vi "Touch_Board.vi"() -> ()   [LabVIEW 2013]
uses:
  <resource>/objmgr/IMAQImage.rc
  <vilib>/vision/NI_Vision_Development_Module.lvlib
  User32.dll
  <vilib>/userdefined/High Color/IMAQdx.ctl
panel:
  in  "NEXT":bool
  in  "Boolean 2":bool
  out "x-y":sgl
  in  "Boolean":bool
  out "Increment":dbl
  in  "reset":i32(listbox)
  in  "Screen Resolution":cluster{"x":i32, "y":i32}={"x"=1366, "y"=768}
  out "Image Size":cluster{"x":i32, "y":i32}
  in  "stop":bool
  in  "Main Tab":enum32{"Page 1", "Page 2"}(tab)
  out "Image":T1(plugin-control)
  in  "Control Panel Tab":enum32{"Page 1", "Page 2", "Page 3"}(tab)
  out "Processed FPS":dbl(knob) scale=0.0..100.0
  out "Acquired FPS":dbl(knob) scale=0.0..100.0 scale format="%.1f"
  in  "Camera Name":T2="cam8"
  out "Buffer No.":u32=4294967295
  in  "Pulse":bool=TRUE
  in  "roi":bool
  in  "mask":bool
  in  "creat calib":bool
  in  "IR":bool
  in  "detect":bool
  in  "touch points":bool
  in  "open calib":bool
  in  "calc":bool=TRUE
  in  "cursor":bool=TRUE
  in  "Click":bool
  in  "Start":bool
  in  "Step":i32
  in  "Settings Tab":T3(tab)=enum."auto calib"
  in  "Prompt":string="Select The Rectangle - Screen Rregion"
  in  "Rectangle":T4 {"Rotation" format="%.2f"; "Left" scale=0.0..1024.0; "Right" scale=0.0..1024.0}
  in  "Color Palette":u32(colorbox)
  in  "ROI Descriptor":T5={"Global Rectangle"=[161, 85, 600, 422], "Contours"=[{"ID"=enum."External", "Type"=3, "Coordinates"=[161, 85, 600, 422]}]} {"Contours"."Type" items=["No Selection", "Point", "Line", "Rectangle", "Oval", "Polygon", "Free", "Annulus", "Unused2", "Unused3", "Broken Line", "Free Hand Line", "Rotated Rectangle"]}
  in  "Out / In":bool
  in  "Shrink":bool=TRUE
  out "Rect Array":i32[](array[numeric])
  in  "Camera Position":u16(ring)
  out "Q":dbl
  in  "Path":path=path "I:/Works/NI/Gesture/Touch Board/TB/cam.png"
  in  "Reference Points":T6 {"Unit" items=["Undefined", "Angstrom", "micrometer", "millimeter", "centimeter", "meter", "kilometer", "microinch", "inch", "feet", "nautic miles", "standard miles", "steps"]; "Real World Coordinates"."Y" format="%.2f"; "Real World Coordinates"."X" format="%.2f"; "Pixel Coordinates"."Y" format="%.2f"; "Pixel Coordinates"."X" format="%.2f"}
  in  "Calibration Axis Info":T7={"Origin Pixel"={"X"=0.0, "Y"=0.0}, "Angle Relative to Horizontal (deg)"=0.0, "Axis Reference"=1} {"Axis Reference" items=["Direct", "Indirect"]; "Angle Relative to Horizontal (deg)" format="%.2f"; "Origin Pixel"."Y" format="%.2f"; "Origin Pixel"."X" format="%.2f"}
  in  "Calibration Learn Setup":T8 {"Corrected Image Learn ROI" items=["Full Image ", "Calibration ROI", "ROI", "Calibration AND ROI", "Calibration OR ROI"]; "Corrected Image Scaling" items=["Scale to Preserve Area", "Scale to Fit"]; "Distortion" items=["Perspective", "Nonlinear"]}
  in  "Point":dbl
  out "Screen Points":T9={"R1"={"x"=0, "y"=0}, "R2"={"x"=1365, "y"=0}, "R3"={"x"=1365, "y"=767}, "R4"={"x"=0, "y"=767}}
  in  "R4":cluster{"x":i32, "y":i32}={"x"=0, "y"=767}
  in  "R3":cluster{"x":i32, "y":i32}={"x"=1365, "y"=767}
  in  "R2":cluster{"x":i32, "y":i32}={"x"=1365, "y"=0}
  in  "R1":cluster{"x":i32, "y":i32}
  in  "Path 2":path=path "I:/Works/NI/Gesture/Touch Board/TB/cam.png"
  in  "Interpolation Type":u32(ring)=1 items=["Zero Order", "Bi-Linear", "Quadratic", "Cubic Spline"]
  in  "Color Plane":i32(ring) items=["Red", "Green", "Blue", "Hue", "Saturation", "Luminance", "Value", "Intensity"]
  in  "Low Pass/High Pass (Low)":bool
  in  "Square/Hexa (Square)":bool
  in  "Connectivity 4/8 (8)":bool=TRUE
  in  "Number of Erosion":i32=1
  in  "Range":cluster{"Lower value":sgl, "Upper value":sgl}={"Lower value"=80.78014, "Upper value"=255.0} {"Lower value" scale=0.0..255.0; "Upper value" scale=0.0..255.0}
  in  "Connectivity 4/8 (8) 2":bool=TRUE
  out "Detect?":bool
  in  "ROI Side":T10={"Global Rectangle"=[0], "Contours"=[{"ID"=enum."External", "Type"=3, "Coordinates"=[]}]} {"Contours"."Type" items=["No Selection", "Point", "Line", "Rectangle", "Oval", "Polygon", "Freehand Region", "Annulus", "Unused2", "Unused3", "Broken Line", "Freehand Line", "Rotated Rectangle"]}
  in  "Settings S":T11={"Contrast"=1, "Filter width"=4, "Steepness"=2, "Subsampling Ratio"=5, "Show Search Area"=TRUE, "Show Search Lines"=TRUE, "Show Edges Found"=TRUE, "Show Result"=TRUE}
  in  "Settings T":T11={"Contrast"=1, "Filter width"=4, "Steepness"=2, "Subsampling Ratio"=5, "Show Search Area"=TRUE, "Show Search Lines"=TRUE, "Show Edges Found"=TRUE, "Show Result"=TRUE}
  out "Distance T":sgl format="%.2f"
  out "Distance S":sgl format="%.2f"
  in  "ROI Top":T10={"Global Rectangle"=[], "Contours"=[{"ID"=enum."External", "Type"=3, "Coordinates"=[]}]} {"Contours"."Type" items=["No Selection", "Point", "Line", "Rectangle", "Oval", "Polygon", "Freehand Region", "Annulus", "Unused2", "Unused3", "Broken Line", "Freehand Line", "Rotated Rectangle"]}
  out "Points of Contact T":cluster{"X":sgl, "Y":sgl}[](array[cluster]) {"Y" format="%.2f"; "X" format="%.2f"}
  out "Points of Contact S":cluster{"X":sgl, "Y":sgl}[](array[cluster]) {"Y" format="%.2f"; "X" format="%.2f"}
  in  "Scanning axis S":u32(ring) items=["Horizontal", "Vertical"]
  in  "Scanning axis T":u32(ring)=1 items=["Horizontal", "Vertical"]
  out "Centre":cluster{"X":sgl, "Y":sgl}
  out "Object Origin":cluster{"X":sgl, "Y":sgl}
  in  "Kx":dbl
  in  "Ky":dbl
  in  "C4":cluster{"x":i16, "y":i16}
  in  "C3":cluster{"x":i16, "y":i16}
  in  "C2":cluster{"x":i16, "y":i16}
  in  "C1":cluster{"x":i16, "y":i16}
  in  "Shift Origin":dbl
  out "Original":bool
  in  "Pulse Width":u32=50
  out "Delay":bool
  out "Stop Pulse":bool
  out "Start Pulse":bool
  in  "Screen Origin":cluster{"x":i16, "y":i16}
  out "M X":dbl
  out "M Y":dbl
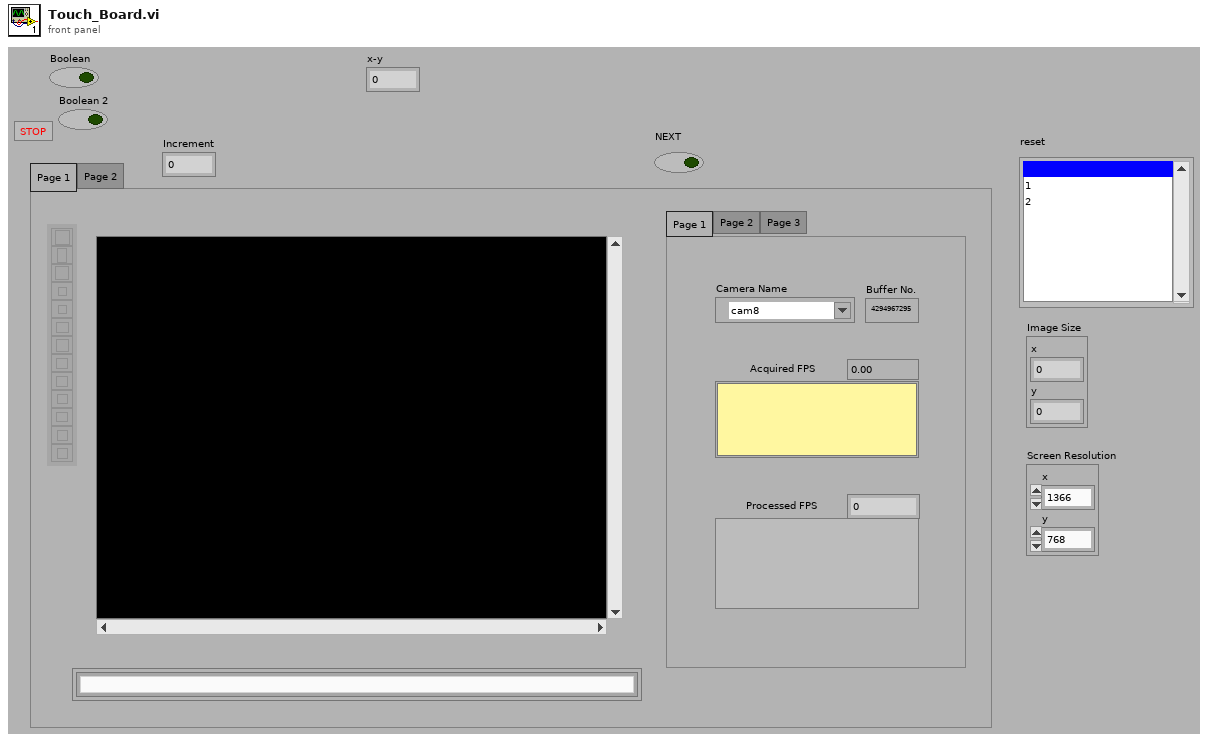
[diagram p1: front panel]
types:
  T1 = typedef "IMAQ Image.ctl" = refnum<image>
  T2 = typedef "IMAQdx.ctl" = refnum<k21>
  T3 = enum32{"rect", "mask", "creat calib", "open calib", "image process", "detect", "calc", "pulse", "Cursor", "auto calib"}
  T4 = typedef "IMAQ Rectangle" = cluster{"Left":i32, "Top":i32, "Right":i32, "Bottom":i32, "Rotation":dbl}
  T5 = cluster{"Global Rectangle":i32[], "Contours":cluster{"ID":enum32{"External", "Internal"}, "Type":u32, "Coordinates":i32[]}[]}
  T6 = cluster{"Pixel Coordinates":cluster{"X":sgl, "Y":sgl}[], "Real World Coordinates":cluster{"X":sgl, "Y":sgl}[], "Unit":u32}
  T7 = cluster{"Origin Pixel":cluster{"X":sgl, "Y":sgl}, "Angle Relative to Horizontal (deg)":sgl, "Axis Reference":u32}
  T8 = cluster{"Distortion":sgl, "Corrected Image Scaling":sgl, "Corrected Image Learn ROI":sgl, "Learn Error Map?":bool, "Learn Correction Table?":bool}
  T9 = cluster{"R1":cluster{"x":i16, "y":i16}, "R2":cluster{"x":i16, "y":i16}, "R3":cluster{"x":i16, "y":i16}, "R4":cluster{"x":i16, "y":i16}}
  T10 = typedef "ROI Descriptor" = cluster{"Global Rectangle":i32[], "Contours":cluster{"ID":enum32{"External", "Internal"}, "Type":u32, "Coordinates":i32[]}[]}
  T11 = cluster{"Contrast":i32, "Filter width":i32, "Steepness":i32, "Subsampling Ratio":u32, "Show Search Area":bool, "Show Search Lines":bool, "Show Edges Found":bool, "Show Result":bool}
  T12 = cluster{"Left":i32, "Top":i32, "Right":i32, "Bottom":i32}
  T13 = cluster{"Height":i32, "Height":i32, "x":i32, "y":i32}
  T14 = cluster{"R1":cluster{"x":i32, "y":i32}, "R2":cluster{"x":i32, "y":i32}, "R3":cluster{"x":i32, "y":i32}, "R4":cluster{"x":i32, "y":i32}}
  T15 = cluster{"Value":cluster{"x":i32, "y":i32}, cluster{"x":i32, "y":i32}, "Value":cluster{"x":i32, "y":i32}, "Value":cluster{"x":i32, "y":i32}}
  T16 = cluster{"Angles (deg)[0]":sgl, "Angles (deg)[1]":sgl, "Angles (deg)[2]":sgl, "Angles (deg)[3]":sgl, "Angles (deg)[4]":sgl, "Angles (deg)[5]":sgl, "Angles (deg)[6]":sgl, "Angles (deg)[7]":sgl, "Angles (deg)[8]":sgl}
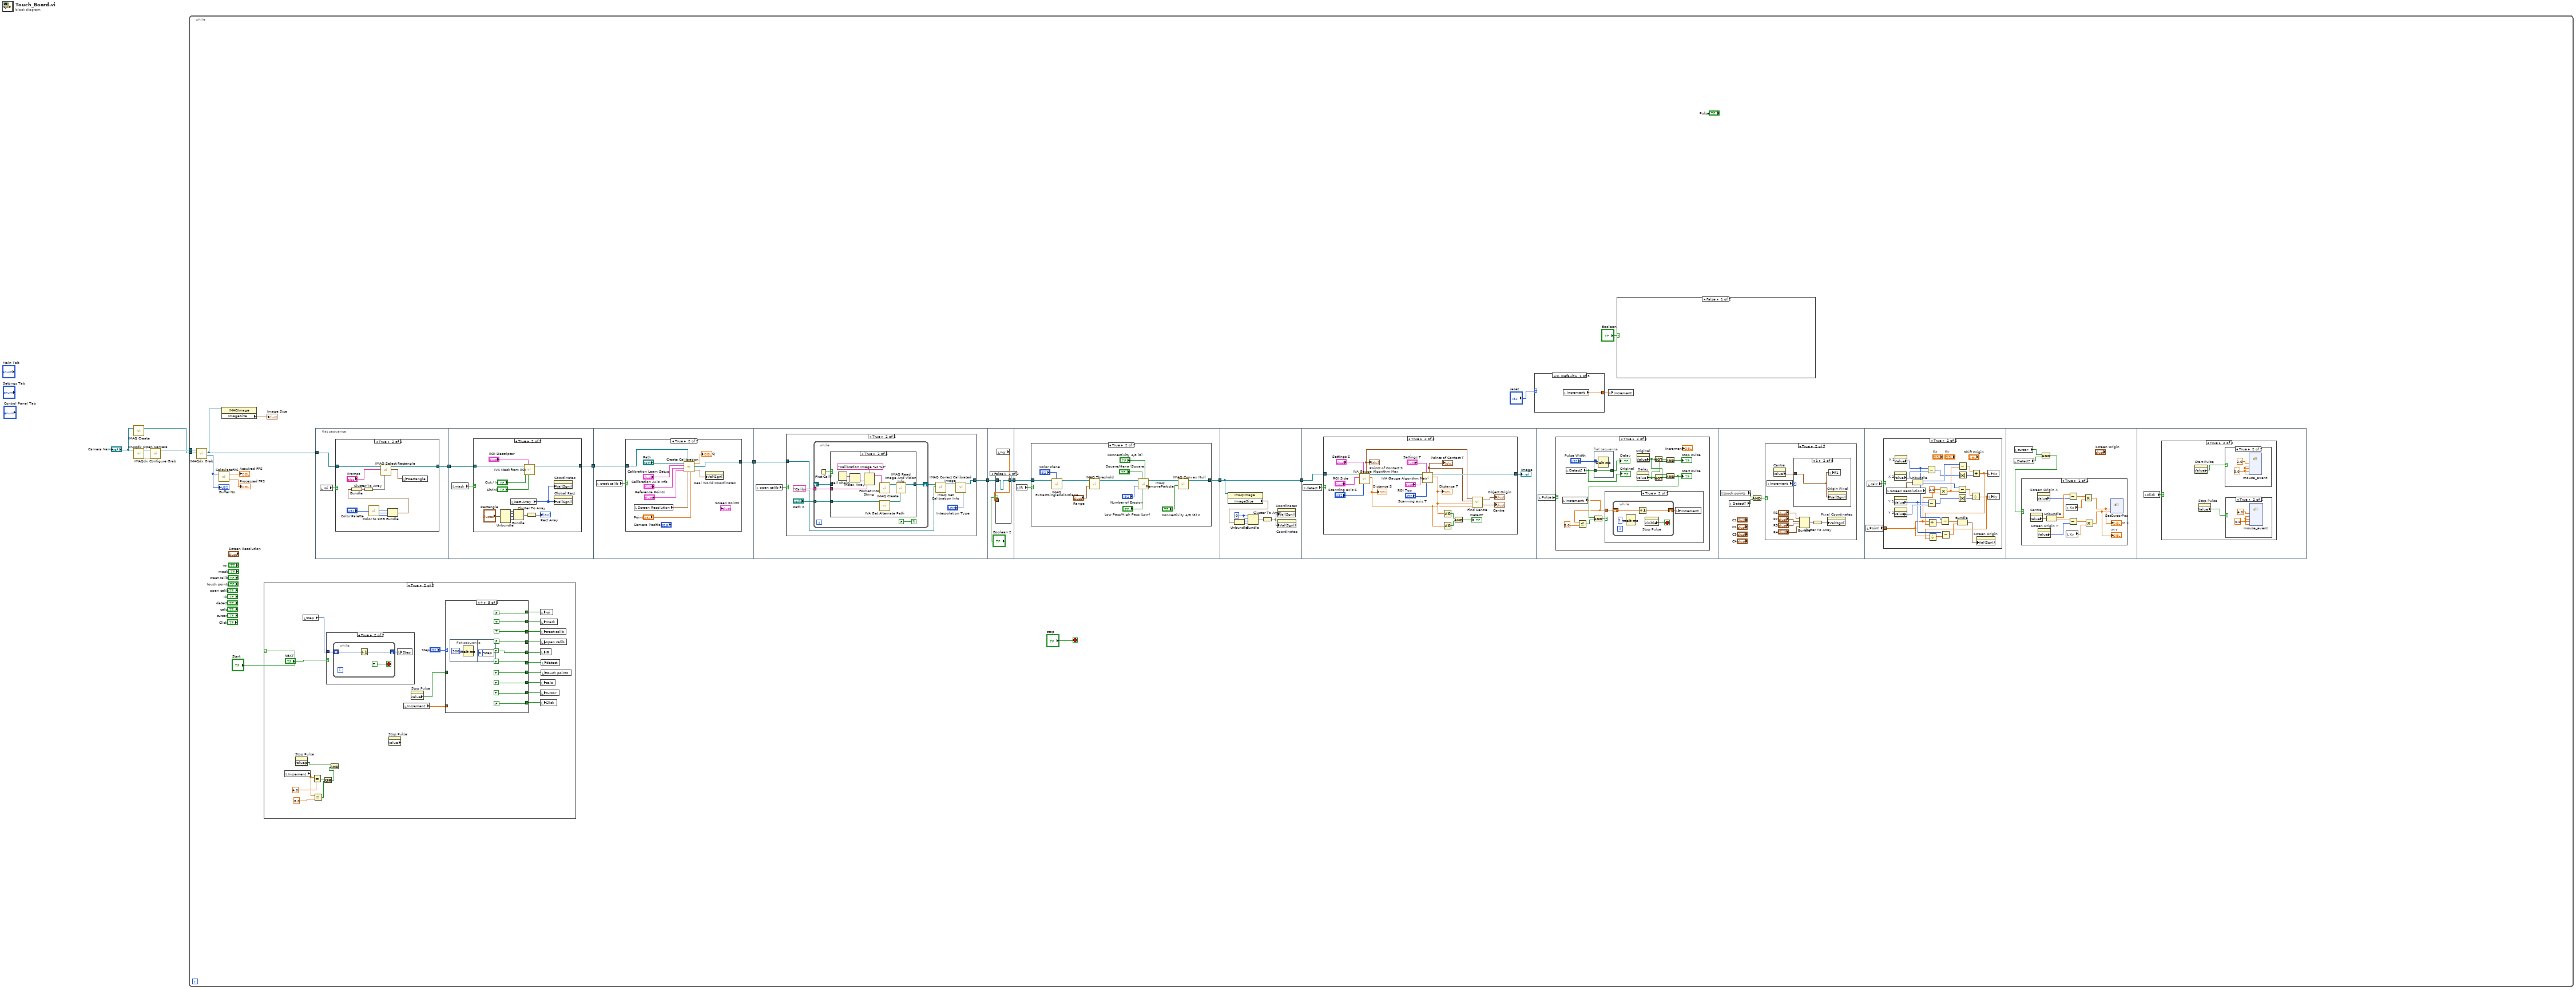
[diagram p0: block diagram]
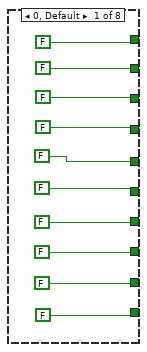
[diagram p4: hidden frame]
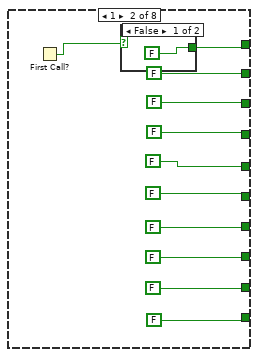
[diagram p5: hidden frame]
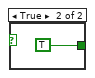
[diagram p6: hidden frame]
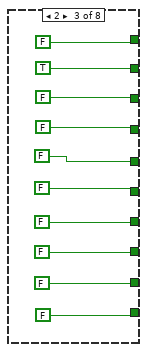
[diagram p7: hidden frame]
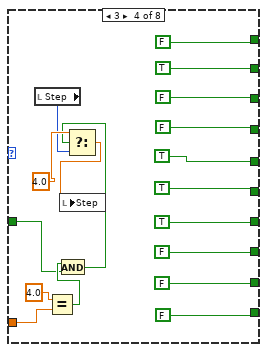
[diagram p8: hidden frame]
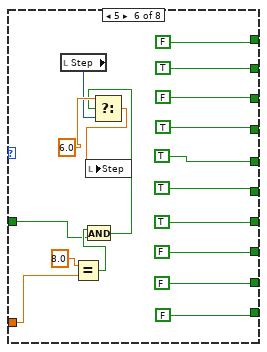
[diagram p9: hidden frame]
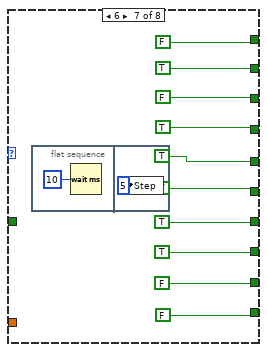
[diagram p10: hidden frame]
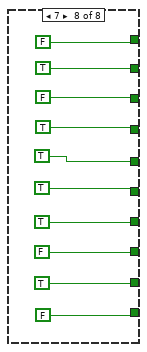
[diagram p11: hidden frame]
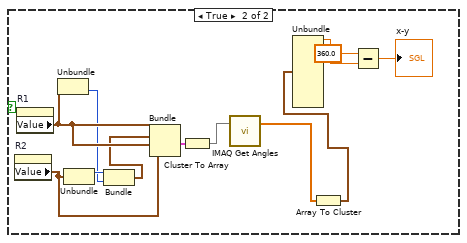
[diagram p12: hidden frame]
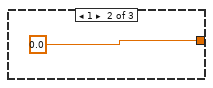
[diagram p13: hidden frame]
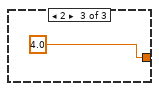
[diagram p14: hidden frame]
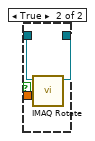
[diagram p20: hidden frame]
diagram:
  n1 = call "IMAQ Create"("Image Name"="Camera Name") -> ("New Image"=w1:T1)  [unwired: 3 in, 2 out]
  n2 = call <vilib>:"IMAQdx Open Camera.vi"("Session In"="Camera Name") -> ("error out"=w4:errorcluster, "Session Out"=w3:T2)  [unwired: 2 in, 7 out]
  n3 = call <vilib>:"IMAQdx Configure Grab.vi"("error in"=w4, "Session In"=w3) -> ("Session Out"=w2:T2)  [unwired: 8 in, 1 out]
  n4 = while {
    tunnel: w2 -> [w24]
    tunnel: w1 -> [w23]
    stop <- "stop" stop-if-true
    n5 = call <vilib>:"IMAQdx Grab.vi"("Image In"=w23, "Session In"=w24) -> ("Buffer Number Out"=w22:u32, "Image Out"=w15:T1)  [unwired: 2 in, 6 out]
    "Buffer No." <- w22
    n6 = call "CalculateFPS.vi"("buffer number"=w22) -> ("processed FPS"=→"Processed FPS":dbl, "acquired FPS"=→"Acquired FPS":dbl)  [unwired: 1 out]
    n7 = property class="IMAQImage"(reference=w15) -> ("ImageSize"=→"Image Size":cluster{"x":i32, "y":i32})  [unwired: 1 in, 2 out]
    n8 = case shown="True" "Start" {
      frame False {
      }
      frame True {
        n9 = local read "Increment"() -> (w30:dbl)
        n10 = property on="Stop Pulse" class="Bool (strict)"() -> ("Value"=w34:bool)  [unwired: 2 in, 2 out]
        n11 = local read "Step"() -> (w43:i32)
        n12 = Equal?(x=w30, y=4.0) -> (x = y?=w32:bool)
        n13 = Equal?(x=w30, y=8.0) -> (x = y?=w31:bool)
        n14 = Or(x=w32, y=w31) -> (x .or. y?=w28:bool)
        n15 = case shown="True" "NEXT" {
          tunnel: w43 -> [_ w47]
          frame False {
          }
          frame True {
            n16 = while {
              shift-right: [w49] -> w48
              shift-left: w47 -> [w50]
              stop <- TRUE stop-if-true
              n17 = Increment(x=w50) -> (x+1=w49:i32)
            }
            n18 = local write "Step"(w48) -> ()
          }
        }
        n19 = And(x=w34, y=w28) -> ()  [unwired: 1 out]
        n20 = property on="Stop Pulse" class="Bool (strict)" props=["Value"]() -> ()  [unwired: 2 in, 3 out]
        n21 = local read "Increment"() -> (w25:dbl)
        n22 = property on="Stop Pulse" class="Bool (strict)"() -> ("Value"=w26:bool)  [unwired: 2 in, 2 out]
        n23 = case shown="4" "Step" {
          tunnel: [FALSE w72 FALSE FALSE FALSE FALSE FALSE FALSE] -> w46
          tunnel: [FALSE FALSE TRUE TRUE TRUE TRUE TRUE TRUE] -> w45
          tunnel: [FALSE FALSE FALSE FALSE TRUE FALSE FALSE FALSE] -> w44
          tunnel: [FALSE FALSE FALSE FALSE FALSE TRUE TRUE TRUE] -> w41
          tunnel: [FALSE FALSE FALSE TRUE FALSE TRUE TRUE TRUE] -> w40
          tunnel: [FALSE FALSE FALSE TRUE FALSE TRUE TRUE TRUE] -> w36
          tunnel: [FALSE FALSE FALSE TRUE FALSE TRUE TRUE TRUE] -> w35
          tunnel: [FALSE FALSE FALSE FALSE FALSE FALSE TRUE FALSE] -> w39
          tunnel: [FALSE FALSE FALSE FALSE FALSE FALSE FALSE TRUE] -> w38
          tunnel: [FALSE FALSE FALSE FALSE FALSE FALSE FALSE FALSE] -> w37
          tunnel: w26 -> [_ _ _ w89 _ w115 _ _]
          tunnel: w25 -> [_ _ _ w92 _ w116 _ _]
          frame 0, Default {
          }
          frame 1 {
            n24 = First Call?() -> (First Call?: T/F=w62:bool)
            n25 = case shown="False" w62 {
              tunnel: [FALSE TRUE] -> w72
              frame False {
              }
              frame True {
              }
            }
          }
          frame 2 {
          }
          frame 3 {
            n26 = local read "Step"() -> (w86:i32)
            n27 = Equal?(x=4.0 ("y"), y=w92) -> (x = y?=w90:bool)
            n28 = And(x=w90, y=w89) -> (x .and. y?=w85:bool)
            n29 = Select(t=4.0 ("y"), s=w85, f=w86) -> (s? t:f=w87:dbl)
            n30 = local write "Step"(w87) -> ()
          }
          frame 4 {
            n31 = flat-sequence {
              frame #0 {
                n32 = Wait (ms)(milliseconds to wait=u32 500) -> ()  [unwired: 1 out]
              }
              frame #1 {
                n33 = local write "Step"(5 ("Step")) -> ()
              }
            }
          }
          frame 5 {
            n34 = local read "Step"() -> (w118:i32)
            n35 = Equal?(x=8.0 ("y"), y=w116) -> (x = y?=w121:bool)
            n36 = And(x=w121, y=w115) -> (x .and. y?=w117:bool)
            n37 = Select(t=6.0 ("y"), s=w117, f=w118) -> (s? t:f=w119:dbl)
            n38 = local write "Step"(w119) -> ()
          }
          frame 6 {
            n39 = flat-sequence {
              frame #0 {
                n40 = Wait (ms)(milliseconds to wait=u32 10) -> ()  [unwired: 1 out]
              }
              frame #1 {
                n41 = local write "Step"(5 ("Step")) -> ()
              }
            }
          }
          frame 7 {
          }
        }
        n42 = local write "roi"(w46) -> ()
        n43 = local write "mask"(w45) -> ()
        n44 = local write "creat calib"(w44) -> ()
        n45 = local write "open calib"(w41) -> ()
        n46 = local write "IR"(w40) -> ()
        n47 = local write "calc"(w39) -> ()
        n48 = local write "cursor"(w38) -> ()
        n49 = local write "Click"(w37) -> ()
        n50 = local write "detect"(w36) -> ()
        n51 = local write "touch points"(w35) -> ()
      }
    }
    n52 = flat-sequence {
      tunnel: w15 -> [w171]
      tunnel: [w172] -> w18
      tunnel: w18 -> [w187]
      tunnel: [w186] -> w17
      tunnel: w17 -> [w204]
      tunnel: [w203] -> w14
      tunnel: w14 -> [w218]
      tunnel: [w216] -> w8
      tunnel: w8 -> [w246]
      tunnel: [w245] -> w7
      tunnel: w7 -> [w252]
      tunnel: [w251] -> w13
      tunnel: w13 -> [w267]
      tunnel: [w267] -> w12
      tunnel: w12 -> [w275]
      frame #0 {
        n53 = local read "roi"() -> (w170:bool)
        n54 = case shown="True" w170 {
          tunnel: [w173 w176] -> w172
          tunnel: w171 -> [w173 w175]
          frame False {
          }
          frame True {
            n55 = call <vilib>:"Color to RGB.vi"("Color"="Color Palette") -> ("R"=w183:u8, "G"=w182:u8, "B"=w181:u8)  [unwired: 1 out]
            n56 = Bundle("R"=w183, "G"=w182, "B"=w181) -> (w179:cluster{"R":u8, "G":u8, "B":u8})  [unwired: 1 in]
            n57 = Bundle(w179) -> (w178:cluster{cluster{"R":u8, "G":u8, "B":u8}})  [unwired: 1 in]
            n58 = Cluster To Array(cluster=w178) -> (array=w180:cluster{"R":u8, "G":u8, "B":u8}[])
            n59 = call "IMAQ Select Rectangle"("Color Palette"=w180, "Prompt"="Prompt", "Image In"=w175) -> ("Rectangle"=w177:T4, "Image Out (duplicate)"=w176:T1)  [unwired: 5 in, 2 out]
            n60 = local write "Rectangle"(w177) -> ()
          }
        }
      }
      frame #1 {
        n61 = local read "mask"() -> (w185:bool)
        n62 = case shown="True" w185 {
          tunnel: w187 -> [w188 w200]
          tunnel: [w188 w190] -> w186
          frame False {
          }
          frame True {
            n63 = Unbundle("Rectangle") -> ("Left"=w197:i32, "Top"=w196:i32, "Right"=w194:i32, "Bottom"=w195:i32)  [unwired: 1 out]
            n64 = local read "Rect Array"() -> (w189:i32[])
            n65 = Bundle("Left"=w197, "Top"=w196, "Right"=w194, "Bottom"=w195) -> (w193:T12)  [unwired: 1 in]
            n66 = call <vilib>:"IVA Mask from ROI.vi"("Shrink"="Shrink", "ROI Descriptor"="ROI Descriptor", "Out / In"="Out / In", "Image Src"=w200) -> ("Image Out"=w190:T1)  [unwired: 1 in, 6 out]
            n67 = Cluster To Array(cluster=w193) -> (array=→"Rect Array":i32[])
            n68 = property on="Coordinates" class="Arr (strict)"("Val(Sgnl)"=w189) -> ()  [unwired: 2 in, 2 out]
            n69 = property on="Global Rect" class="Arr (strict)"("Val(Sgnl)"=w189) -> ()  [unwired: 2 in, 2 out]
          }
        }
      }
      frame #2 {
        n70 = local read "creat calib"() -> (w202:bool)
        n71 = case shown="True" w202 {
          tunnel: w204 -> [w205 w215]
          tunnel: [w205 w206] -> w203
          frame False {
          }
          frame True {
            n72 = local read "Screen Resolution"() -> (w210:cluster{"x":i32, "y":i32})
            n73 = call "Create Calibration.vi"("Point Value"="Point", "Screen Resolution"=w210, "Reference Points"="Reference Points", "Calibration Axis Info"="Calibration Axis Info", "Image"=w215, "Calibration Learn Setup"="Calibration Learn Setup", "Path"="Path") -> ("Screen Points"=w207:cluster{"Point Value":sgl, "Point Value":sgl}[], "Image Out (duplicate)"=w206:T1, "Quality Score"=→"Q":sgl)  [unwired: 1 in]
            n74 = property on="Real World Coordinates" class="Arr (strict)"("Val(Sgnl)"=w207) -> ()  [unwired: 2 in, 2 out]
          }
        }
      }
      frame #3 {
        n75 = local read "open calib"() -> (w217:bool)
        n76 = case shown="True" w217 {
          tunnel: w218 -> [w219 w221]
          tunnel: [w219 w220] -> w216
          frame False {
          }
          frame True {
            n77 = while "Load the calibrated image and apply the calibration to the source image." {
              shift-right: [w231] -> w224
              shift-left: _ -> [w230]
              tunnel: "Path 2" -> [w228]
              tunnel: "Calibration from Image 1" ("Step Name") -> [w227]
              stop <- FALSE continue-if-true
              n78 = First Call?() -> (First Call?: T/F=w232:bool)
              n79 = case shown="True" w232 {
                tunnel: [w233 w240] -> w231
                tunnel: w230 -> [w233 _]
                tunnel: w228 -> [_ w236]
                tunnel: w227 -> [_ w234]
                frame False {
                }
                frame True {
                  n80 = Call Chain() -> (call chain=w238:string[])
                  n81 = Index Array(array=w238) -> (element=w237:string)  [unwired: 1 in]
                  n82 = Format Into String(format string="Calibration Image %s %s" ("Image Name"), w237, w234) -> (resulting string=w242:string)  [unwired: 2 in, 1 out]
                  n83 = call "IMAQ Create"("Image Name"=w242) -> ("New Image"=w239:T1)  [unwired: 3 in, 2 out]
                  n84 = call <vilib>:"IVA Get Alternate Path.vi"("Path In"=w236) -> ("Path Out"=w235:path)  [unwired: 10 out]
                  n85 = call "IMAQ Read Image And Vision Info"("File Path"=w235, "Image"=w239) -> ("Image Out"=w240:T1)  [unwired: 2 in, 7 out]
                }
              }
            }
            n86 = call "IMAQ Set Calibration Info"("Image Dst"=w221, "Image Src"=w224) -> ("Calibrated Image"=w223:T1)  [unwired: 2 in, 7 out]
            n87 = call "IMAQ Correct Calibrated Image"("Interpolation Type"="Interpolation Type", "Image Src"=w223) -> ("Corrected Image"=w220:T1)  [unwired: 5 in, 4 out]
          }
        }
      }
      frame #4 {
        n88 = local read "x-y"() -> (w244:sgl)
        n89 = case shown="False" "Boolean 2" {
          tunnel: w246 -> [w247 w250]
          tunnel: [w247 w249] -> w245
          tunnel: w244 -> [_ w248]
          frame False {
          }
          frame True {
            n90 = call "IMAQ Rotate"("Angle (degrees)"=w248, "Image Src"=w250) -> ("Image Dst Out"=w249:T1)  [unwired: 8 in, 1 out]
          }
        }
      }
      frame #5 {
        n91 = local read "IR"() -> (w253:bool)
        n92 = case shown="True" w253 {
          tunnel: [w254 w256] -> w251
          tunnel: w252 -> [w254 w255]
          frame False {
          }
          frame True {
            n93 = call "IMAQ ExtractSingleColorPlane"("Color Plane"="Color Plane", "Image Src"=w255) -> ("Image Dst Out"=w263:T1)  [unwired: 2 in, 7 out]
            n94 = call "IMAQ Threshold"("Range"="Range", "Image Src"=w263) -> ("Image Dst Out"=w265:T1)  [unwired: 4 in, 5 out]
            n95 = call "IMAQ RemoveParticle"("Connectivity 4/8 (8)"="Connectivity 4/8 (8)", "Low Pass/High Pass (Low)"="Low Pass/High Pass (Low)", "Square/Hexa (Square)"="Square/Hexa (Square)", "Number of Erosion"="Number of Erosion", "Image Src"=w265) -> ("Image Dst Out"=w266:T1)  [unwired: 2 in, 4 out]
            n96 = call "IMAQ Convex Hull"("Connectivity 4/8 (8)"="Connectivity 4/8 (8) 2", "Image Src"=w266) -> ("Image Dst Out"=w256:T1)  [unwired: 2 in, 7 out]
          }
        }
      }
      frame #6 {
        w268 = 0 ("Height")
        n97 = property class="IMAQImage"(reference=w267) -> ("ImageSize"=w272:cluster{"x":i32, "y":i32})  [unwired: 1 in, 2 out]
        n98 = Unbundle(w272) -> ("x"=w269:i32, "y"=w270:i32)
        n99 = Bundle("Height"=w268, "Height"=w268, "x"=w269, "y"=w270) -> (w271:T13)  [unwired: 1 in]
        n100 = Cluster To Array(cluster=w271) -> (array=w273:i32[])
        n101 = property on="Coordinates" class="Arr (strict)"("Val(Sgnl)"=w273) -> ()  [unwired: 2 in, 2 out]
        n102 = property on="Coordinates" class="Arr (strict)"("Val(Sgnl)"=w273) -> ()  [unwired: 2 in, 2 out]
      }
      frame #7 {
        n103 = local read "detect"() -> (w276:bool)
        n104 = case shown="True" w276 {
          tunnel: w275 -> [w277 w293]
          tunnel: [w277 w287] -> w274
          frame False {
          }
          frame True {
            n105 = call <vilib>:"IVA Gauge Algorithm Max.vi"("Scanning axis"="Scanning axis S", "Settings"="Settings S", "ROI Descriptor"="ROI Side", "Image"=w293) -> ("Distance"=w281:sgl, "Image Out"=w288:T1, "Points of Contact"=w284:cluster{"X":sgl, "Y":sgl}[])  [unwired: 2 in, 3 out]
            "Distance S" <- w281
            "Points of Contact S" <- w284
            n106 = call <vilib>:"IVA Gauge Algorithm Max.vi"("Scanning axis"="Scanning axis T", "Settings"="Settings T", "ROI Descriptor"="ROI Top", "Image"=w288) -> ("Distance"=w282:sgl, "Image Out"=w287:T1, "Points of Contact"=w283:cluster{"X":sgl, "Y":sgl}[])  [unwired: 2 in, 3 out]
            "Distance T" <- w282
            "Points of Contact T" <- w283
            n107 = Not Equal To 0?(x=w282) -> (x != 0?=w280:bool)
            n108 = Not Equal To 0?(x=w281) -> (x != 0?=w279:bool)
            n109 = And(x=w280, y=w279) -> (x .and. y?=→"Detect?":bool)
            n110 = call "Find Centre.vi"("Top Distance"=w281, "Side Distance"=w282, "Top Edge Point"=w283, "Side Edge Point"=w284) -> ("Centre"=→"Centre":cluster{"X":sgl, "Y":sgl}, "Object Origin"=→"Object Origin":cluster{"X":sgl, "Y":sgl})
          }
        }
        "Image" <- w274
      }
      frame #8 {
        n111 = local read "Pulse"() -> (w296:bool)
        n112 = case shown="True" w296 {
          frame False {
          }
          frame True {
            n113 = local read "Increment"() -> (w297:dbl)
            n114 = local read "Detect?"() -> (w307:bool)
            "Original" <- w307
            n115 = Less Or Equal?(x=w297, y=8.0) -> (x <= y?=w298:bool)
            n116 = flat-sequence {
              tunnel: w307 -> [w317]
              tunnel: [w317] -> w309
              tunnel: "Pulse Width" -> [w316]
              frame #0 {
                n117 = Wait (ms)(milliseconds to wait=w316) -> ()  [unwired: 1 out]
              }
            }
            n118 = property on="Delay" class="Bool (strict)"() -> ("Value"=w302:bool)  [unwired: 2 in, 2 out]
            n119 = property on="Original" class="Bool (strict)"() -> ("Value"=w303:bool)  [unwired: 2 in, 2 out]
            n120 = Not(x=w303) -> (.not. x?=w305:bool)
            n121 = Not(x=w302) -> (.not. x?=w304:bool)
            n122 = And(x=w305, y=w302) -> (x .and. y?=→"Stop Pulse":bool)
            n123 = And(x=w303, y=w304) -> (x .and. y?=w300:bool)
            "Start Pulse" <- w300
            n124 = And(x=w300, y=w298) -> (x .and. y?=w301:bool)
            n125 = case shown="True" w301 {
              tunnel: w297 -> [_ w310]
              frame False {
              }
              frame True {
                n126 = while {
                  shift-right: [w313] -> w311
                  shift-left: w310 -> [w314]
                  stop <- w315 stop-if-true
                  n127 = Wait (ms)(milliseconds to wait=u32 1) -> ()  [unwired: 1 out]
                  n128 = Increment(x=w314) -> (x+1=w313:dbl)
                  n129 = property on="Stop Pulse" class="Bool (strict)"() -> ("Visible"=w315:bool)  [unwired: 2 in, 2 out]
                }
                n130 = local write "Increment"(w311) -> ()
              }
            }
            "Delay" <- w309
          }
        }
      }
      frame #9 {
        n131 = local read "touch points"() -> (w320:bool)
        n132 = local read "Detect?"() -> (w319:bool)
        n133 = And(x=w320, y=w319) -> (x .and. y?=w318:bool)
        n134 = case shown="True" w318 {
          frame False {
          }
          frame True {
            n135 = local read "Increment"() -> (w322:dbl)
            n136 = property on="Centre" class="Clust (strict)"() -> ("Value"=w321:cluster{"X":sgl, "Y":sgl})  [unwired: 2 in, 2 out]
            n137 = case shown="1" w322 {
              tunnel: w321 -> [_ w329 w330 w331 w332 w333 w334 w335 w336]
              frame 0, Default {
              }
              frame 1 {
                n138 = property on="Origin Pixel" class="Clust (strict)"("Val(Sgnl)"=w329) -> ()  [unwired: 2 in, 2 out]
                n139 = local write "R1"(w329) -> ()
              }
              frame 2 {
                n140 = local write "R2"(w330) -> ()
              }
              frame 3 {
                n141 = local write "R3"(w331) -> ()
              }
              frame 4 {
                n142 = local write "R4"(w332) -> ()
              }
              frame 5 {
                n143 = local write "C1"(w333) -> ()
              }
              frame 6 {
                n144 = local write "C2"(w334) -> ()
              }
              frame 7 {
                n145 = local write "C3"(w335) -> ()
              }
              frame 8 {
                n146 = local write "C4"(w336) -> ()
              }
            }
            n147 = Bundle("R1"="R1", "R2"="R2", "R3"="R3", "R4"="R4") -> (w328:T14)  [unwired: 1 in]
            n148 = Cluster To Array(cluster=w328) -> (array=w325:cluster{"x":i32, "y":i32}[])
            n149 = property on="Pixel Coordinates" class="Arr (strict)"("Val(Sgnl)"=w325) -> ()  [unwired: 2 in, 2 out]
          }
        }
      }
      frame #10 {
        n150 = local read "Point"() -> (w337:dbl)
        n151 = local read "calc"() -> (w338:bool)
        n152 = case shown="True" w338 {
          tunnel: w337 -> [_ w339]
          frame False {
          }
          frame True {
            n153 = local read "Screen Resolution"() -> (w361:cluster{"x":i32, "y":i32})
            n154 = property on="X 2" class="DigNum (strict)"() -> ("Value"=w352:i16)  [unwired: 2 in, 2 out]
            n155 = property on="Y 1" class="DigNum (strict)"() -> ("Value"=w347:i16)  [unwired: 2 in, 2 out]
            n156 = property on="Y 2" class="DigNum (strict)"() -> ("Value"=w351:i16)  [unwired: 2 in, 2 out]
            n157 = property on="X 1" class="DigNum (strict)"() -> ("Value"=w349:i16)  [unwired: 2 in, 2 out]
            n158 = Unbundle(w361) -> ("x"=w356:i32, "y"=w355:i32)
            n159 = Subtract(x=w349, y=w352) -> (x-y=w354:i16)
            n160 = Subtract(x=w347, y=w351) -> (x-y=w353:i16)
            n161 = Multiply(x=2.0, y=w339) -> (x*y=w341:dbl)
            n162 = Subtract(x=w355, y=w341) -> (x-y=w357:dbl)
            n163 = Absolute Value(x=w353) -> (abs(x)=w358:i16)
            n164 = Subtract(x=w356, y=w341) -> (x-y=w360:dbl)
            n165 = Absolute Value(x=w354) -> (abs(x)=w359:i16)
            n166 = Divide(x=w357, y=w358) -> (x/y=w342:dbl)
            n167 = Divide(x=w339, y=w342) -> (x/y=w348:dbl)
            n168 = Subtract(x=w347, y=w348) -> (x-y=w345:dbl)
            n169 = Divide(x=w360, y=w359) -> (x/y=w343:dbl)
            n170 = Divide(x=w339, y=w343) -> (x/y=w350:dbl)
            n171 = Subtract(x=w349, y=w350) -> (x-y=w346:dbl)
            n172 = Bundle(w346, w345) -> (w344:cluster{dbl, dbl})  [unwired: 1 in]
            n173 = property on="Screen Origin" class="Clust (strict)"("Val(Sgnl)"=w344) -> ()  [unwired: 2 in, 2 out]
            n174 = local write "Kx"(w343) -> ()
            n175 = local write "Ky"(w342) -> ()
          }
        }
      }
      frame #11 {
        n176 = local read "Detect?"() -> (w363:bool)
        n177 = local read "cursor"() -> (w364:bool)
        n178 = And(x=w364, y=w363) -> (x .and. y?=w362:bool)
        n179 = case shown="True" w362 {
          frame True {
            n180 = property on="Centre" class="Clust (strict)"() -> ("Value"=w375:cluster{"X":sgl, "Y":sgl})  [unwired: 2 in, 2 out]
            n181 = property on="Screen Origin X" class="DigNum (strict)"() -> ("Value"=w366:i16)  [unwired: 2 in, 2 out]
            n182 = property on="Screen Origin Y" class="DigNum (strict)"() -> ("Value"=w365:i16)  [unwired: 2 in, 2 out]
            n183 = Unbundle(w375) -> ("X"=w374:sgl, "Y"=w373:sgl)
            n184 = local read "Kx"() -> (w370:dbl)
            n185 = local read "Ky"() -> (w369:dbl)
            n186 = Subtract(x=w374, y=w366) -> (x-y=w372:sgl)
            n187 = Subtract(x=w373, y=w365) -> (x-y=w371:sgl)
            n188 = Multiply(x=w372, y=w370) -> (x*y=w368:dbl)
            "M X" <- w368
            n189 = Multiply(x=w371, y=w369) -> (x*y=w367:dbl)
            "M Y" <- w367
            n190 = dll-call lib="user32.dll" fn="SetCursorPos"("dx"=w368, "dy"=w367) -> ()  [unwired: 6 in, 2 out]
          }
          frame False {
          }
        }
      }
      frame #12 {
        n191 = local read "Click"() -> (w376:bool)
        n192 = case shown="True" w376 {
          frame False {
          }
          frame True {
            n193 = property on="Start Pulse" class="Bool (strict)"() -> ("Value"=w377:bool)  [unwired: 2 in, 2 out]
            n194 = property on="Stop Pulse" class="Bool (strict)"() -> ("Value"=w378:bool)  [unwired: 2 in, 2 out]
            n195 = case shown="True" w377 {
              frame False {
                w383 = 0.0 ("Numeric 2")
                n196 = dll-call lib="user32.dll" fn="mouse_event"("dwFlags"=0.0 ("Numeric 2"), "dx"=w383, "dy"=w383, "dwData"=w383, "dwExtraInfo"=w383) -> ()  [unwired: 9 in, 2 out]
              }
              frame True {
                w385 = 0.0 ("Numeric 2")
                n197 = dll-call lib="user32.dll" fn="mouse_event"("dwFlags"=2.0 ("Numeric 2"), "dx"=w385, "dy"=w385, "dwData"=w385, "dwExtraInfo"=w385) -> ()  [unwired: 9 in, 2 out]
              }
            }
            n198 = case shown="True" w378 {
              frame False {
                w379 = 0.0 ("Numeric 2")
                n199 = dll-call lib="user32.dll" fn="mouse_event"("dwFlags"=0.0 ("Numeric 2"), "dx"=w379, "dy"=w379, "dwData"=w379, "dwExtraInfo"=w379) -> ()  [unwired: 9 in, 2 out]
              }
              frame True {
                w381 = 0.0 ("Numeric 2")
                n200 = dll-call lib="user32.dll" fn="mouse_event"("dwFlags"=4.0 ("Numeric 2"), "dx"=w381, "dy"=w381, "dwData"=w381, "dwExtraInfo"=w381) -> ()  [unwired: 9 in, 2 out]
              }
            }
          }
        }
      }
    }
    n201 = case shown="0, Default" "reset" {
      tunnel: [w167 0.0 ("Increment") 4.0 ("Increment")] -> w10
      frame 0, Default {
        n202 = local read "Increment"() -> (w167:dbl)
      }
      frame 1 {
      }
      frame 2 {
      }
    }
    n203 = local write "Increment"(w10) -> ()
    n204 = case shown="False" "Boolean" {
      frame False {
      }
      frame True {
        n205 = property on="R2" class="Clust (strict)"() -> ("Value"=w162:cluster{"x":i32, "y":i32})  [unwired: 2 in, 2 out]
        n206 = property on="R1" class="Clust (strict)"() -> ("Value"=w166:cluster{"x":i32, "y":i32})  [unwired: 2 in, 2 out]
        n207 = Unbundle(w166) -> ("y"=w164:i32)  [unwired: 1 out]
        n208 = Unbundle(w162) -> ("x"=w165:i32)  [unwired: 1 out]
        n209 = Bundle("x"=w165, "y"=w164) -> (w163:cluster{"x":i32, "y":i32})  [unwired: 1 in]
        n210 = Bundle("Value"=w166, w163, "Value"=w166, "Value"=w162) -> (w161:T15)  [unwired: 1 in]
        n211 = Cluster To Array(cluster=w161) -> (array=w160:cluster{"x":i32, "y":i32}[])
        n212 = call "IMAQ Get Angles"("Points"=w160) -> ("Angles (deg)"=w159:sgl[])  [unwired: 4 in, 2 out]
        n213 = Array To Cluster(array=w159) -> (cluster=w158:T16)
        n214 = Unbundle(w158) -> ("Angles (deg)[0]"=w157:sgl)  [unwired: 8 out]
        n215 = Subtract(x=sgl 360.0, y=w157) -> (x-y=→"x-y":sgl)
      }
    }
  }
